vi "general_param.vi"() -> ()   [LabVIEW 2018]
panel:
  in  "工作波长（nm）":u32=400 min=400 max=1100
  in  "编号":string
  in  "激光器型号":string
  # "通用参数"
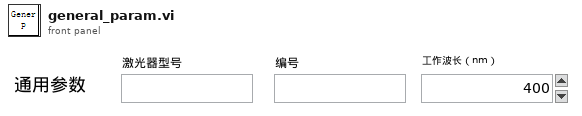
[diagram p1: front panel]
types:
  T1 = cluster{"激光器型号":string, "X":dbl, "Y":dbl, "Z":dbl, "Rotate":dbl, "Pitching":dbl}
  T2 = typedef "IMAQ Image.ctl" = refnum<image>
  T3 = cluster{"示波器":cluster{"Channel (0:Channel 1)":enum16{"Channel 1", "Channel 2", "Channel 3", "Channel 4"}, "电压范围":dbl, "触发电压":dbl, "时间范围":dbl, " 示波器VISA":refnum<visa-resource-name>, "时间范围 标签":u64, "电压范围 标签":u64, "触发电压 标签":u64}, "光谱仪":cluster{"Channel (0:Channel 1)":enum16{"Channel 1", "Channel 2", "Channel 3", "Channel 4"}, "电压范围":u64, "触发电压":u64, "时间范围":u64}, " 近场相机":cluster{"曝光时间":i32, "模拟增益":i32, "控制套接字":i32, "IP 地址":string, " 采集套接字":i32, "  版本号":i32, "ImageData":T2, "  增益最大":i32, "  增益最小":i32, " 曝光最大":i32, " 曝光最小":i32, " 帧速":i32, " 同步切换":i32, "  曝光缩放":i32}, " 偏振仪":cluster{"电压范围":u64, "触发电压":u64, "时间范围":u64, "波长范围":enum16{"可见光 400-700nm", "近红外 700-1100nm"}}, " 功率计":cluster{"通道":enum16{"Channel 1", "Channel 2"}, "工作波长":u32, "单位":u64, "时间范围":u64, "IP地址":string, "端口":u32}, "能量计":cluster{"通道":enum16{"Channel 1", "Channel 2"}, "工作波长":u32, "单位":u64, "时间范围":u64, "IP地址":string, "端口":u32, "能量计量程":enum16{"200uJ", "20uJ", "2uJ", "200nJ"}}, "电机":cluster{"Channel (0:Channel 1)":enum16{"Channel 1", "Channel 2", "Channel 3", "Channel 4"}, "电压范围":u64, "触发电压":u64, "时间范围":u64}, " 远场相机":cluster{"曝光时间":i32, "模拟增益":i32, "控制套接字":i32, "IP 地址":string, " 采集套接字":i32, "  版本号":i32, "ImageData":T2, "  增益最大":i32, "  增益最小":i32, " 曝光最大":i32, " 曝光最小":i32, " 帧速":i32, " 同步切换":i32, "  曝光缩放":i32}}
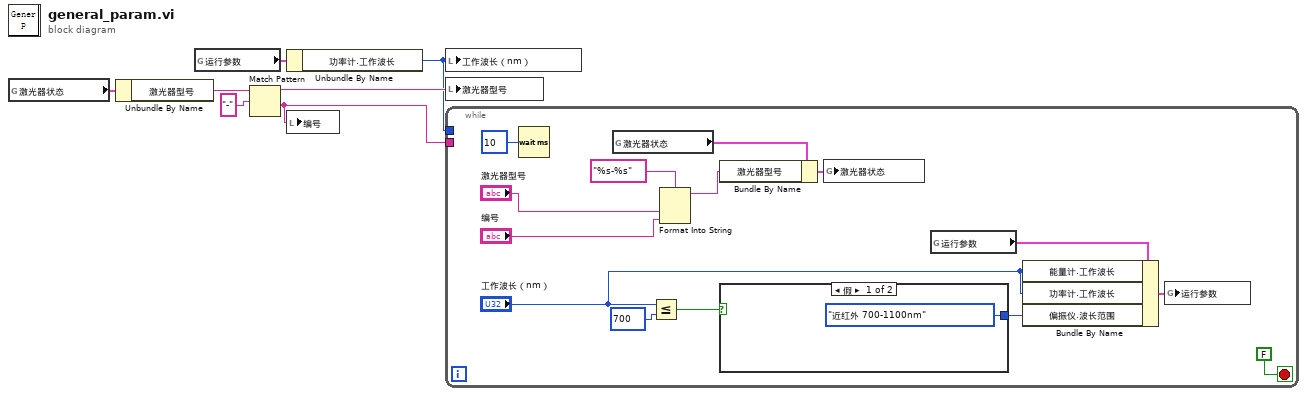
[diagram p0: block diagram]
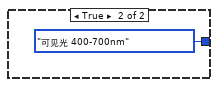
[diagram p2: hidden frame]
diagram:
  n1 = global read "参数.vi" "激光器状态"() -> (w7:T1)
  n2 = Unbundle By Name(w7) -> ("激光器型号"=w6:string)
  n3 = global read "参数.vi" "运行参数"() -> (w3:T3)
  n4 = Match Pattern(string=w6, regular expression="-" ("正则表达式")) -> (before substring=w4:string, after substring=w1:string)  [unwired: 1 in, 2 out]
  n5 = Unbundle By Name(w3) -> ("功率计.工作波长"=w2:u32)
  n6 = local write "编号"(w1) -> ()
  n7 = local write "工作波长（nm）"(w2) -> ()
  n8 = local write "激光器型号"(w4) -> ()
  n9 = while {
    tunnel: w2 -> [_]
    tunnel: w1 -> [_]
    stop <- FALSE stop-if-true
    n10 = Wait (ms)(milliseconds to wait=u32 10 ("等待时间（毫秒）")) -> ()  [unwired: 1 out]
    n11 = global read "参数.vi" "激光器状态"() -> (w16:T1)
    n12 = Less Or Equal?(x="工作波长（nm）", y=u32 700) -> (x <= y?=w12:bool)
    n13 = Format Into String(format string="%s-%s" ("格式字符串"), "激光器型号", "编号") -> (resulting string=w17:string)  [unwired: 2 in, 1 out]
    n14 = Bundle By Name(cluster=w16, "激光器型号"=w17) -> (w19:T1)
    n15 = case shown="假" w12 {
      tunnel: [enum16{"可见光 400-700nm", "近红外 700-1100nm"}."近红外 700-1100nm" ("波长范围") enum16{"可见光 400-700nm", "近红外 700-1100nm"}."可见光 400-700nm" ("波长范围")] -> w11
      frame False {
      }
      frame True {
      }
    }
    n16 = global write "参数.vi" "激光器状态"(w19) -> ()
    n17 = global read "参数.vi" "运行参数"() -> (w15:T3)
    n18 = Bundle By Name(cluster=w15, "能量计.工作波长"="工作波长（nm）", "功率计.工作波长"="工作波长（nm）", "偏振仪.波长范围"=w11) -> (w10:T3)
    n19 = global write "参数.vi" "运行参数"(w10) -> ()
  }
